vi "Keithley2400series_s.vi"() -> ()   [LabVIEW 2014]
uses:
  <vilib>/Utility/file.llb/Write To Spreadsheet File (string).vi
panel:
  in  "Timeout (10000 ms)":i32=10000 format="%#.6g"
  in  "stop":bool
  in  "Source Mode  (0: Voltage)":u16(ring) items=["Voltage", "Current"]
  in  "VISA resource name 2":refnum<visa-resource-name>
  in  "Serial Configuration":T1={"Baud Rate"=9600, "Parity"=0, "Data Bits"=8, "Stop Bits"=10, "Flow Control"=0} {"Flow Control" items=["None", "XON/XOFF", "RTS/CTS", "XON/XOFF & RTS/CTS", "DTR/DSR", "XON/XOFF & DTR/DSR"]; "Stop Bits" items=["1.0"=10, "1.5"=15, "2.0"=20]; "Data Bits" items=["7"=7, "8"=8]; "Parity" items=["None", "Odd", "Even", "Mark", "Space"]; "Baud Rate" items=["300"=300, "600"=600, "1200"=1200, "2400"=2400, "4800"=4800, "9600"=9600, "19200"=19200]}
  in  "Файл записи замеров":path
  in  "Ограничение":dbl format="%.2f"
  out "Замер":string
  in  "Выход":dbl
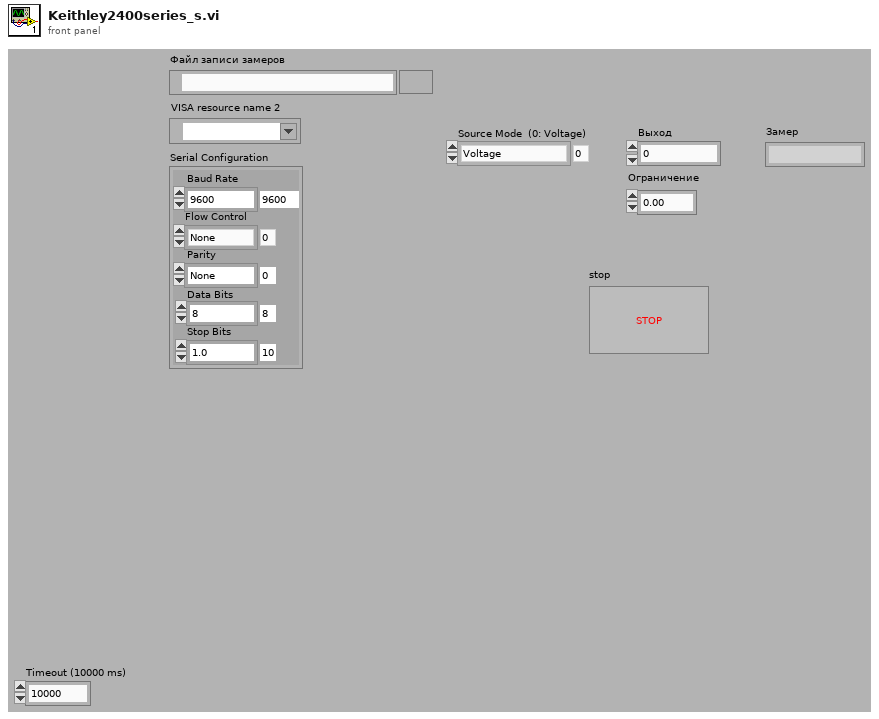
[diagram p1: front panel]
types:
  T1 = cluster{"Baud Rate":u32, "Parity":u16, "Data Bits":u16, "Stop Bits":u16, "Flow Control":u16}
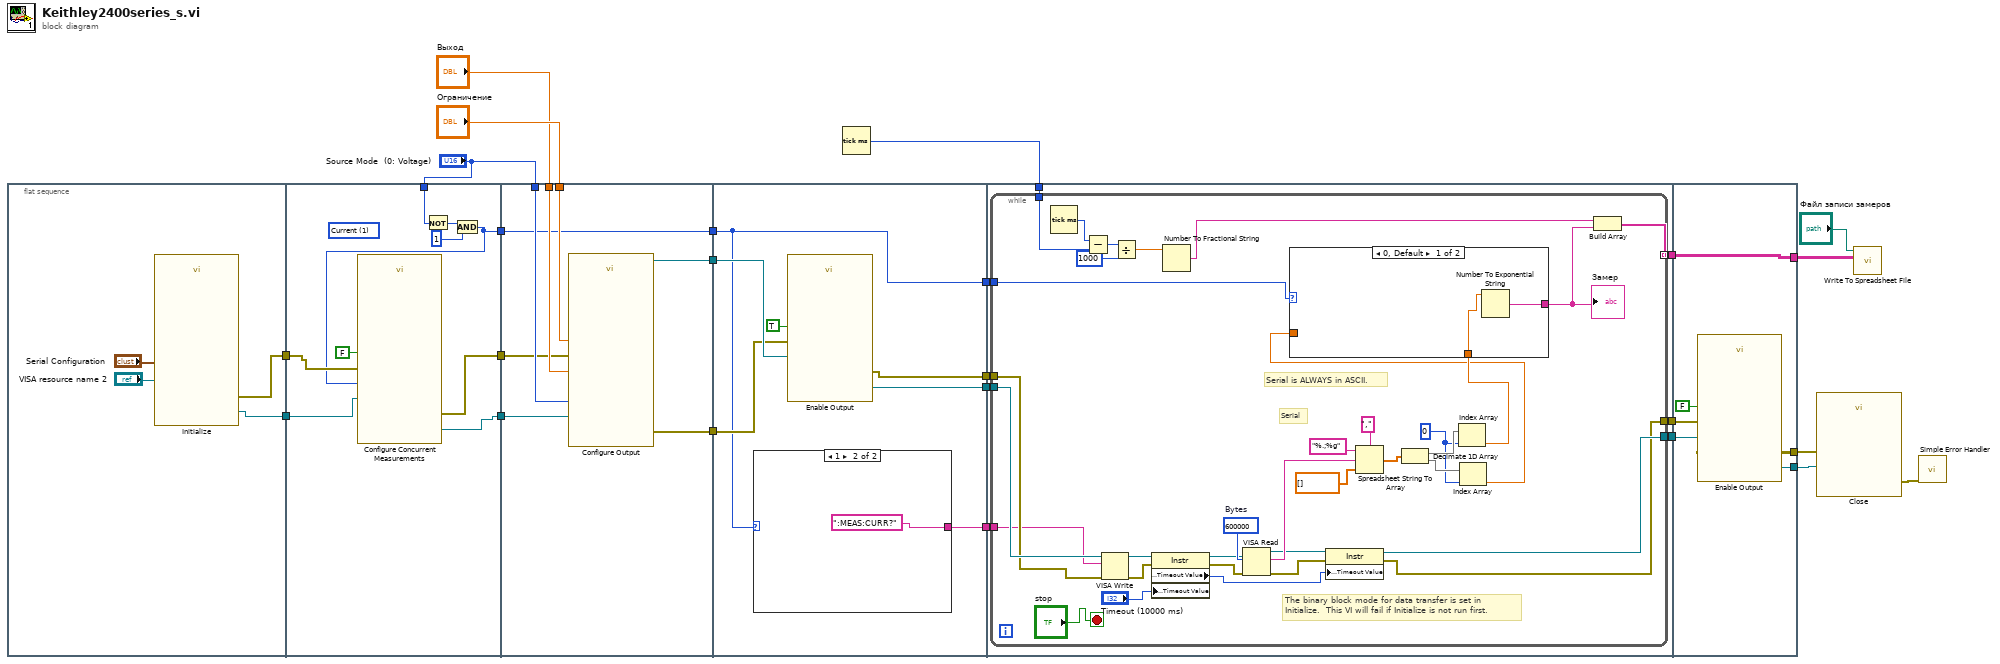
[diagram p0: block diagram]
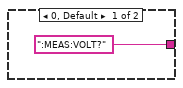
[diagram p2: hidden frame]
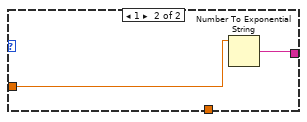
[diagram p3: hidden frame]
diagram:
  n1 = flat-sequence {
    tunnel: [w26] -> w9
    tunnel: [w25] -> w7
    tunnel: w9 -> [w35]
    tunnel: [w36] -> w8
    tunnel: w7 -> [w34]
    tunnel: [w37] -> w6
    tunnel: "Source Mode  (0: Voltage)" -> [w32]
    tunnel: [w29] -> w2
    tunnel: "Ограничение" -> [w45]
    tunnel: "Выход" -> [w44]
    tunnel: "Source Mode  (0: Voltage)" -> [w43]
    tunnel: w8 -> [w42]
    tunnel: w6 -> [w41]
    tunnel: [w40] -> w22
    tunnel: [w39] -> w21
    tunnel: [w38] -> w4
    tunnel: w2 -> [w38]
    tunnel: w22 -> [w52]
    tunnel: w21 -> [w51]
    tunnel: [w49] -> w20
    tunnel: [w48] -> w19
    tunnel: w4 -> [w47]
    tunnel: [w47] -> w3
    tunnel: [w46] -> w1
    tunnel: w20 -> [w62]
    tunnel: w19 -> [w61]
    tunnel: w18 -> [w60]
    tunnel: [w59] -> w15
    tunnel: [w58] -> w14
    tunnel: [w57] -> w13
    tunnel: w3 -> [w56]
    tunnel: w1 -> [w55]
    tunnel: [w106] -> w16
    tunnel: w15 -> [w106]
    tunnel: w14 -> [w104]
    tunnel: w13 -> [w103]
    tunnel: [w102] -> w12
    tunnel: [w101] -> w11
    frame #0 {
      n2 = call "Initialize.vi"("Serial Configuration"="Serial Configuration", "VISA resource name"="VISA resource name 2") -> ("error out"=w25:errorcluster, "VISA resource name out"=w26:refnum<visa-resource-name>)  [unwired: 8 in]
    }
    frame #1 {
      (unwired) u16 1 items=["Volts", "Current", "Resistance", "Volt, Current", "Volts, Resistance", "Current, Resistance", "All"] ("Measurement Selection (3: Volts, Current)")
      n3 = Not(x=w32) -> (.not. x?=w31:u16)
      n4 = And(x=w31, y=u16 1) -> (x .and. y?=w29:u16)
      n5 = call "Configure Concurrent Measurements.vi"("error in (no error)"=w34, "Measurement Selection (3: Volts, Current)"=w29, "Enable Concurrent Measurements (F: Disable)"=FALSE, "VISA resource name"=w35) -> ("error out"=w37:errorcluster, "VISA resource name out"=w36:refnum<visa-resource-name>)  [unwired: 6 in]
    }
    frame #2 {
      n6 = call "Configure Output.vi"("Source Mode  (0: Voltage)"=w43, "error in (no error)"=w41, "Compliance  Level (0.1)"=w45, "Output Level (0)"=w44, "VISA resource name"=w42) -> ("error out"=w39:errorcluster, "VISA resource name out"=w40:refnum<visa-resource-name>)  [unwired: 5 in]
    }
    frame #3 {
      n7 = case shown="1" w47 {
        tunnel: [":MEAS:VOLT?" ":MEAS:CURR?"] -> w46
        frame 0, Default {
        }
        frame 1 {
        }
      }
      n8 = call "Enable Output.vi"("error in (no error)"=w51, "Enable Output (T: Enable)"=TRUE, "VISA resource name"=w52) -> ("error out"=w49:errorcluster, "VISA resource name out"=w48:refnum<visa-resource-name>)  [unwired: 7 in]
    }
    frame #4 {
      n9 = while {
        tunnel: w62 -> [w74]
        tunnel: w61 -> [w75]
        tunnel: w60 -> [w91]
        tunnel: [w89] -> w59 mode=indexing
        tunnel: [w73] -> w58
        tunnel: [w72] -> w57
        tunnel: w56 -> [w65]
        tunnel: w55 -> [w63]
        stop <- "stop" stop-if-true
        w68 = 0 ("index")
        w82 = u32 600000  # Bytes
        # "Serial is ALWAYS in ASCII."
        # "Serial"
        # "The binary block mode for data transfer is set in Initialize.  This VI will fail if Initialize is not run first."
        n10 = Tick Count (ms)() -> (millisecond timer value=w95:u32)
        n11 = Subtract(x=w95, y=w91) -> (x-y=w94:u32)
        n12 = VISA Write(VISA resource name=w75, write buffer=w63, error in (no error)=w74) -> (VISA resource name out=w83:refnum<visa-resource-name>, error out=w76:errorcluster)  [unwired: 1 out]
        n13 = Divide(x=w94, y=u32 1000) -> (x/y=w92:dbl)
        n14 = property class="Instr"(reference=w83, error in=w76, "General Settings:Timeout Value"="Timeout (10000 ms)") -> (reference out=w77:refnum<visa-resource-name>, error out=w78:errorcluster, "General Settings:Timeout Value"=w88:u32)
        n15 = Number To Fractional String(number=w92) -> (F-format string=w90:string)  [unwired: 3 in]
        n16 = VISA Read(VISA resource name=w77, byte count=w82, error in (no error)=w78) -> (VISA resource name out=w80:refnum<visa-resource-name>, read buffer=w87:string, error out=w81:errorcluster)  [unwired: 1 out]
        n17 = property class="Instr"(reference=w80, error in=w81, "General Settings:Timeout Value"=w88) -> (reference out=w73:refnum<visa-resource-name>, error out=w72:errorcluster)
        n18 = Spreadsheet String To Array(delimiter (Tab)=",", format string="%.;%g", spreadsheet string=w87, array type (2D Dbl)=sgl[] []) -> (array=w71:sgl[])
        n19 = Decimate 1D Array(w71) -> (w70:sgl[], w69:sgl[])
        n20 = Index Array(array=w70, index=w68) -> (element=w67:sgl)
        n21 = Index Array(array=w69, index=w68) -> (element=w64:sgl)
        n22 = case shown="0, Default" w65 {
          tunnel: w64 -> [_ w100]
          tunnel: w67 -> [w98 _]
          tunnel: [w97 w99] -> w66
          frame 0, Default {
            n23 = Number To Exponential String(number=w98) -> (E-format string=w97:string)  [unwired: 3 in]
          }
          frame 1 {
            n24 = Number To Exponential String(number=w100) -> (E-format string=w99:string)  [unwired: 3 in]
          }
        }
        "Замер" <- w66
        n25 = Build Array(w90, w66) -> (w89:string[])
      }
    }
    frame #5 {
      n26 = call "Enable Output.vi"("error in (no error)"=w103, "Enable Output (T: Enable)"=FALSE, "VISA resource name"=w104) -> ("error out"=w102:errorcluster, "VISA resource name out"=w101:refnum<visa-resource-name>)  [unwired: 7 in]
    }
  }
  n27 = Tick Count (ms)() -> (millisecond timer value=w18:u32)
  n28 = call "Close.vi"("error in (no error)"=w12, "VISA resource name"=w11) -> ("error out"=w10:errorcluster)  [unwired: 9 in]
  n29 = call-poly <vilib>:"Write To Spreadsheet File.vi"("2D data"=w16, "file path (dialog if empty)"="Файл записи замеров") -> ()  [unwired: 6 in, 1 out]
  n30 = call <vilib>:"Simple Error Handler.vi"("error in (no error)"=w10) -> ()  [unwired: 4 in, 5 out]
